vi "Rsrc.vi"(5 "RF":T2 items=["RF_0", "RF_1", "RF_2", "RF_3"], 7 "RFU":T1, 8 "Error_In":errorcluster, 10 "Auto_Sel_Rsrc?":bool=TRUE, 11 "VISA_Rsrc_In":refnum<visa-resource-name>) -> (0 "Error_Out":errorcluster, 3 "VISA_Rsrc_Out":refnum<visa-resource-name>)   [LabVIEW 2018]
uses:
  Types/RF.ctl
  Types/RFU.ctl
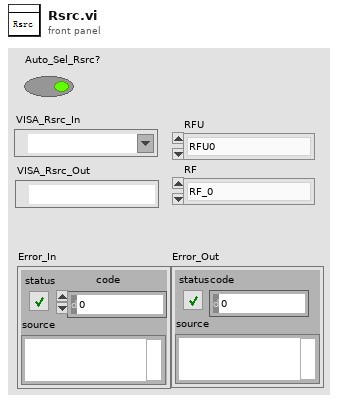
[diagram p1: front panel]
types:
  T1 = typedef "RFU.ctl" = enum8{"RFU0", "RFU1", "RFU2", "RFU3", "RFU4"}
  T2 = typedef "RF.ctl" = u16
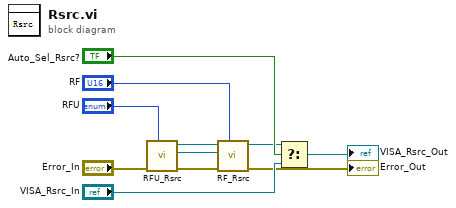
[diagram p0: block diagram]
diagram:
  n1 = call "RFU_Rsrc.vi"("RFU"="RFU", "error in (no error)"="Error_In") -> ("error out"=w4:errorcluster, "K7_1"=w8:refnum<visa-resource-name>, "K7_0"=w9:refnum<visa-resource-name>)  [unwired: 7 in]
  n2 = call "RF_Rsrc.vi"("RF"="RF", "Error_In"=w4, "K7_1"=w8, "K7_0"=w9) -> ("Error_Out"=→"Error_Out":errorcluster, "Rsrc"=w6:refnum<visa-resource-name>)  [unwired: 6 in]
  n3 = Select(t=w6, s="Auto_Sel_Rsrc?", f="VISA_Rsrc_In") -> (s? t:f=→"VISA_Rsrc_Out":refnum<visa-resource-name>)
